vi "Module Type.vi"(11 "GenericGuiAO in":refnum<class "GenericGuiAO.lvclass">) -> (2 "Module Type":string)   [LabVIEW 2020, in "VolatusDAQGenericGUI.lvlib" / "GenericGuiAO.lvclass"]
uses:
  GenericGuiAO.lvclass
  GenericGuiAO.lvclass/GenericGuiAO.ctl
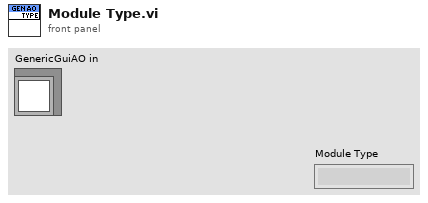
[diagram p1: front panel]
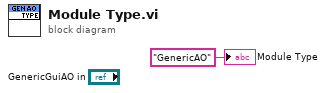
[diagram p0: block diagram]
diagram:
  "Module Type" <- "GenericAO" ("Module Type")
